vi "global-JKISMQFGVChangeTStamp.vi"() -> ()   [LabVIEW 2014, in "JKI-State-Machine-Plus.lvlib"]
uses:
  JKI-State-Machine-Plus.lvlib
panel:
  in  "global-JKISMQFGVChangeTStamp":u32
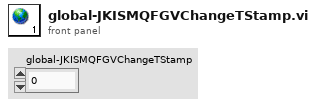
[diagram p1: front panel]
diagram:
